vi "CRYGet Time Curve array.vi"(4 "Scaling":u16=1, 6 "Unit Info In":T5={"Y unit In"="dB", "dB ref In"=1.0, "Y unit Out"="dB", "dB ref Out"=1.0, "Y unit Curve"="dB", "dB ref Curve"=1.0, "Y data  Curve"=0, "Y data Time"=0}, 7 "Additive Info":T2, 8 "Harmonics array":dbl[](array[numeric]), 9 "Option Array In":bool[](array[boolean]), 10 "Averaging":u16, 11 "Algorithm":u16) -> (0 "Display Array":T3(array[cluster]), 1 "Unit Info Out":T4[](array[typedef]), 2 "Curve Info Array Out":T1)   [LabVIEW 2013]
uses:
  Typedef Control/CRYUnit Info Cluster.ctl
  Typedef Control/CRYUnit Info Out Cluster.ctl
  Typedef Control/CRYAnalysis CurveName Cluster.ctl
panel:
  in  "Is Impedance?":bool
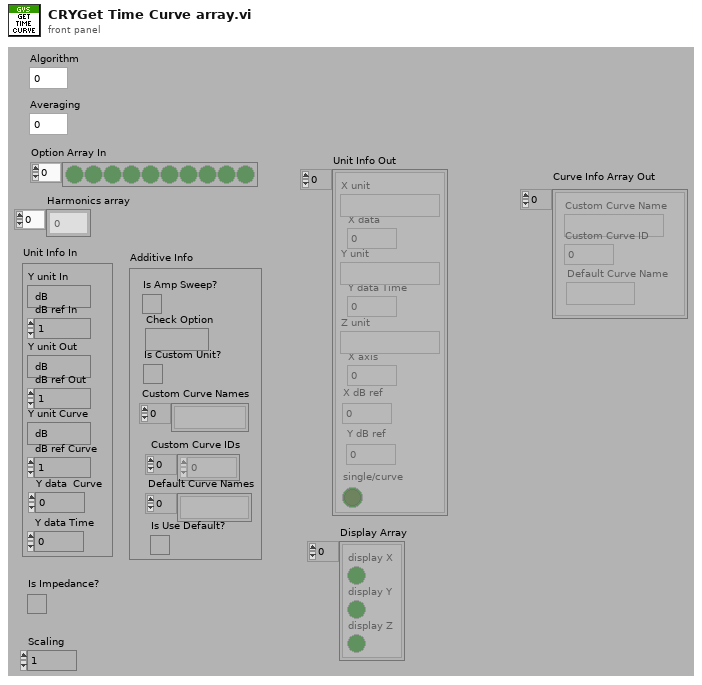
[diagram p1: front panel]
types:
  T1 = typedef "CRYAnalysis CurveName Cluster.ctl" = cluster{"Custom Curve Name":string, "Custom Curve ID":i32, "Default Curve Name":string}[]
  T2 = cluster{"Is Amp Sweep?":bool, "Check Option":string, "Is Custom Unit?":bool, "Custom Curve Names":string[], "Custom Curve IDs":i32[], "Default Curve Names":string[], "Is Use Default?":bool}
  T3 = cluster{"display X":bool, "display Y":bool, "display Z":bool}[]
  T4 = typedef "CRYUnit Info Out Cluster.ctl" = cluster{"X unit":string, "X data":u16, "Y unit":string, "Y data Time":u16, "Z unit":string, "X axis":u16, "X dB ref":dbl, "Y dB ref":dbl, "single/curve":bool}
  T5 = typedef "CRYUnit Info Cluster.ctl" = cluster{"Y unit In":string, "dB ref In":dbl, "Y unit Out":string, "dB ref Out":dbl, "Y unit Curve":string, "dB ref Curve":dbl, "Y data  Curve":u16, "Y data Time":u16}
  T6 = cluster{"display X":bool, "display Y":bool, "display Z":bool}
  T7 = enum32{"English", "Chinese", "Korean", "Japanese", "Russian", "Chinese traditional"}
  T8 = cluster{"X unit":string, "X data":u16, "Y unit In":string, "Scaling":u16, "Z unit":string, "X data":u16, "dB ref In":dbl, "dB ref In":dbl, "display X":bool}
  T9 = cluster{"X unit":string, "X data":u16, string, "Scaling":u16, "Z unit":string, "X data":u16, "dB ref In":dbl, "dB ref In":dbl, "display X":bool}
  T10 = cluster{"X unit":string, "X data":u16, string, "Scaling":u16, "Z unit":string, "X data":u16, "dB ref In":dbl, "dB ref In":dbl, "display X":bool}[]
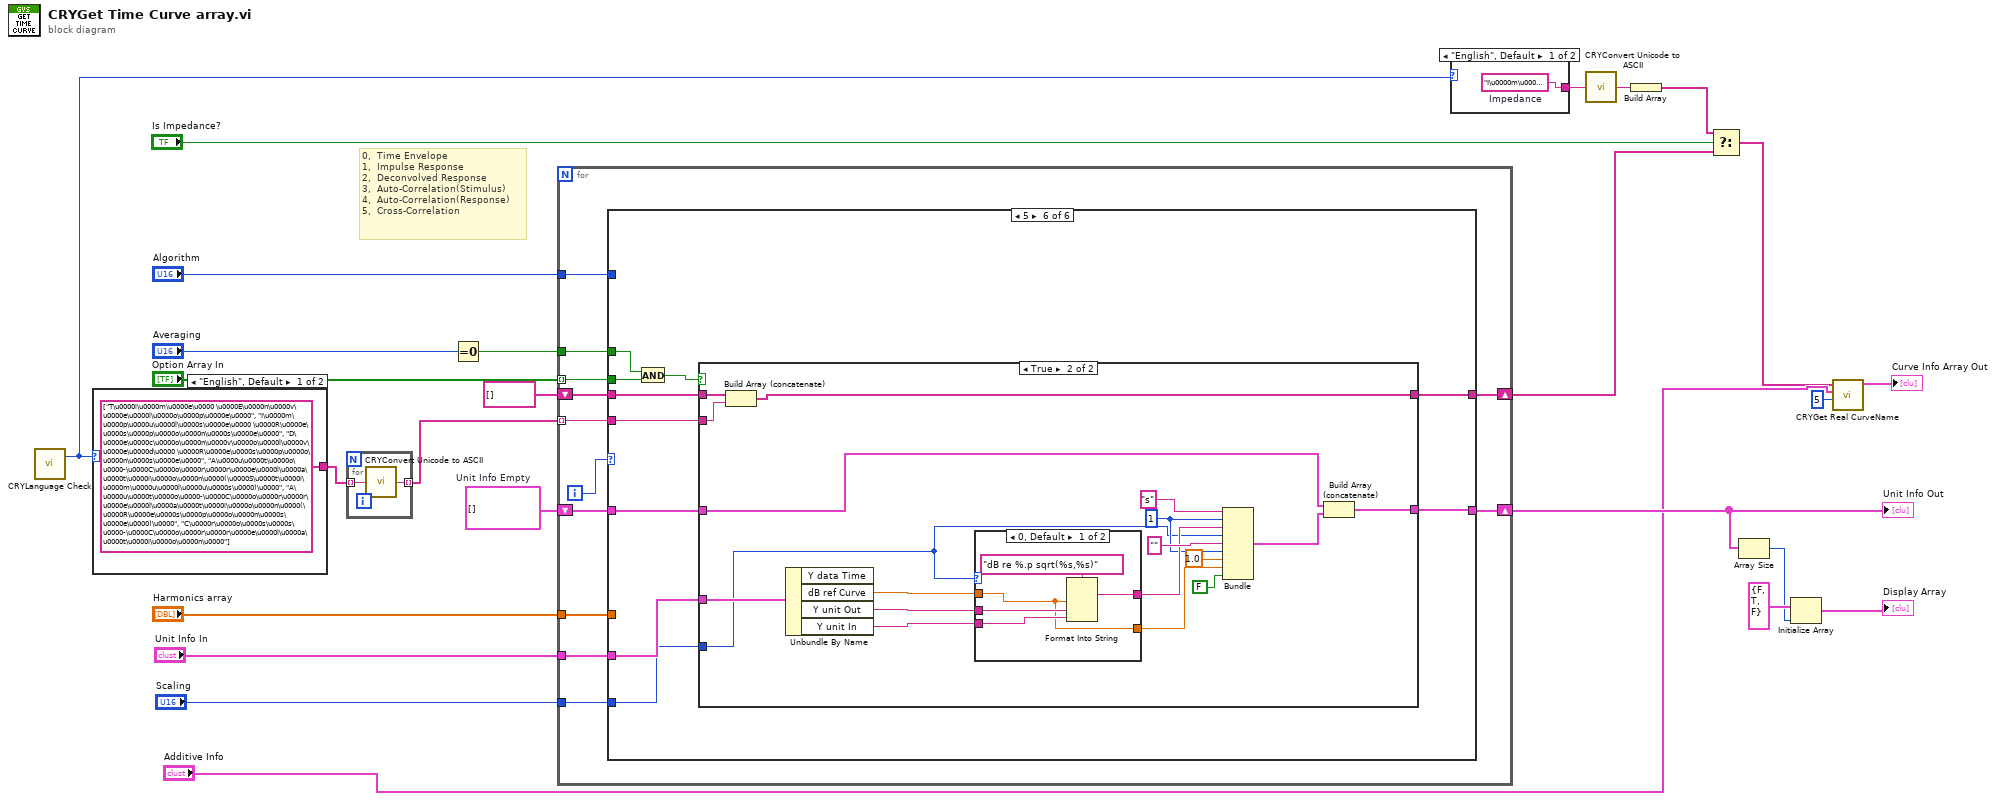
[diagram p0: block diagram]
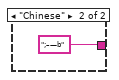
[diagram p2: hidden frame]
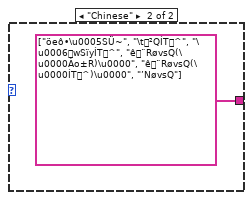
[diagram p3: hidden frame]
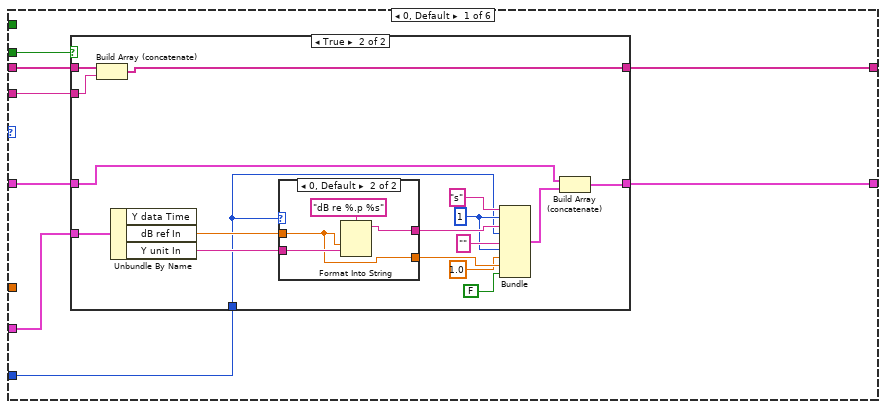
[diagram p4: hidden frame]
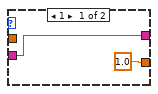
[diagram p6: hidden frame]
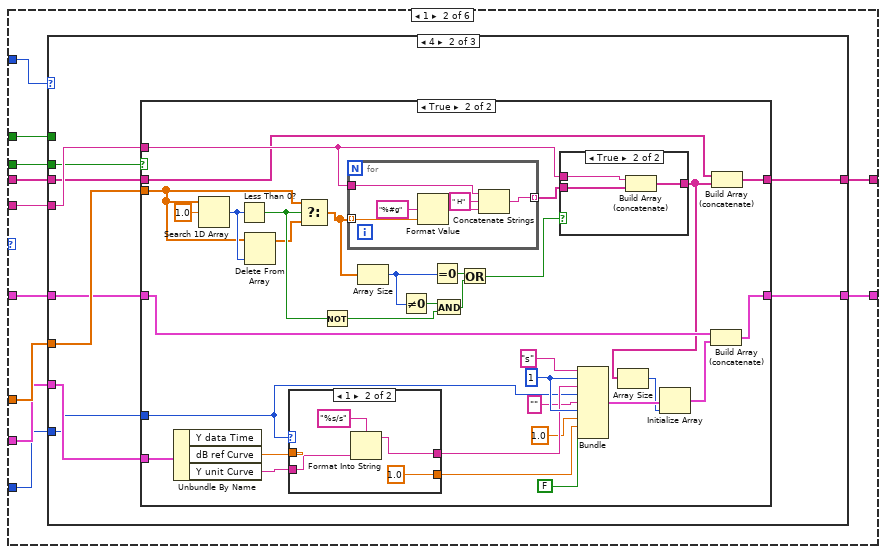
[diagram p7: hidden frame]
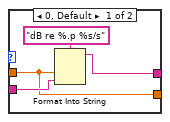
[diagram p10: hidden frame]
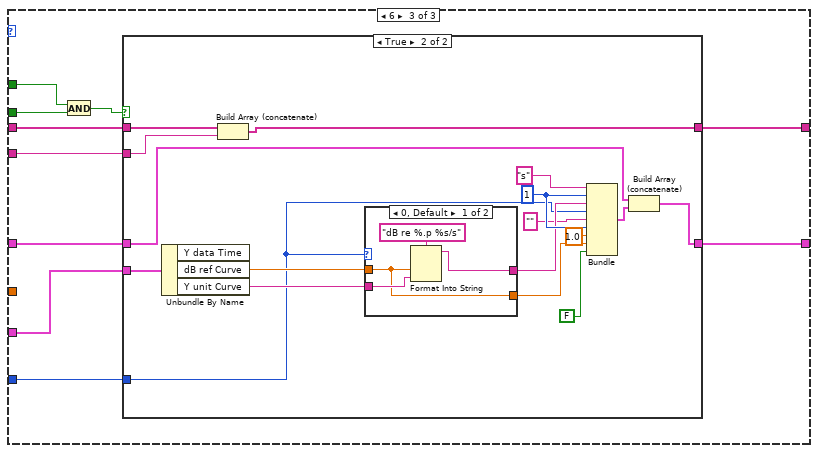
[diagram p12: hidden frame]
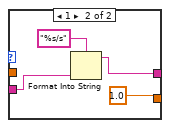
[diagram p14: hidden frame]
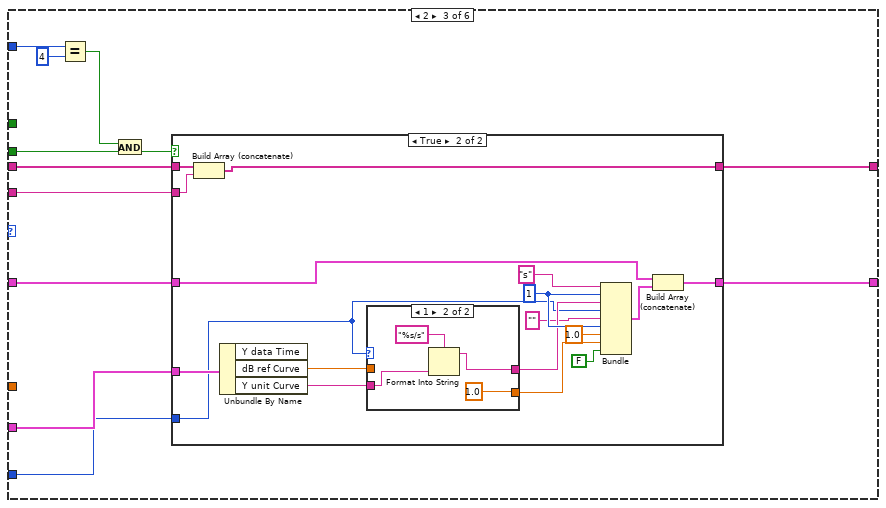
[diagram p15: hidden frame]
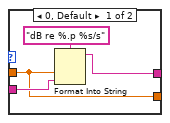
[diagram p17: hidden frame]
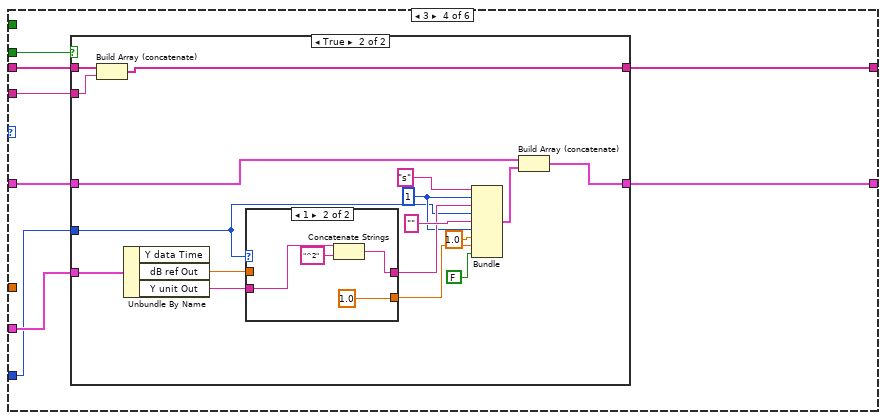
[diagram p18: hidden frame]
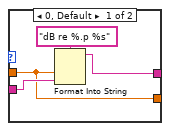
[diagram p20: hidden frame]
diagram:
  w15 = T4[] []  # Unit Info Empty
  # "0,  Time Envelope\n1,  Impulse Response\n2,  Deconvolved Response\n3,  Auto-Correlation(Stimulus)\n4,  Auto-Correlation(Response)\n5,  Cross-Correlation"
  n1 = call "CRYLanguage Check.vi"() -> ("Language"=w1:T7)  [unwired: 10 in, 1 out]
  n2 = case shown="\"English\", Default" w1 {
    tunnel: [string[] ["T\u0000i\u0000m\u0000e\u0000 \u0000E\u0000n\u0000v\u0000e\u0000l\u0000o\u0000p\u0000e\u0000", "I\u0000m\u0000p\u0000u\u0000l\u0000s\u0000e\u0000 \u0000R\u0000e\u0000s\u0000p\u0000o\u0000n\u0000s\u0000e\u0000", "D\u0000e\u0000c\u0000o\u0000n\u0000v\u0000o\u0000l\u0000v\u0000e\u0000d\u0000 \u0000R\u0000e\u0000s\u0000p\u0000o\u0000n\u0000s\u0000e\u0000", "A\u0000u\u0000t\u0000o\u0000-\u0000C\u0000o\u0000r\u0000r\u0000e\u0000l\u0000a\u0000t\u0000i\u0000o\u0000n\u0000(\u0000S\u0000t\u0000i\u0000m\u0000u\u0000l\u0000u\u0000s\u0000)\u0000", "A\u0000u\u0000t\u0000o\u0000-\u0000C\u0000o\u0000r\u0000r\u0000e\u0000l\u0000a\u0000t\u0000i\u0000o\u0000n\u0000(\u0000R\u0000e\u0000s\u0000p\u0000o\u0000n\u0000s\u0000e\u0000)\u0000", "C\u0000r\u0000o\u0000s\u0000s\u0000-\u0000C\u0000o\u0000r\u0000r\u0000e\u0000l\u0000a\u0000t\u0000i\u0000o\u0000n\u0000"] ("Array") string[] ["öeô•\u0005SÜ~", "\t²QÍT^", "\u0006wSïyÍT^", "ê¨RøvsQ(\u0000Ào±R)\u0000", "ê¨RøvsQ(\u0000ÍT^)\u0000", "’NøvsQ"] ("Array")] -> w5
    frame "English", Default {
    }
    frame "Chinese" {
    }
  }
  n3 = for {
    tunnel: w5 -> [w29] mode=indexing
    tunnel: [w28] -> w6 mode=indexing
    n4 = call "CRYConvert Unicode to ASCII.vi"("Unicode"=w29) -> ("ASCII"=w28:string)  [unwired: 4 in]
  }
  n5 = Equal To 0?(x="Averaging") -> (x = 0?=w23:bool)
  n6 = for {
    tunnel: w6 -> [w39] mode=indexing
    tunnel: "Option Array In" -> [w41] mode=indexing
    shift-right: [w38] -> w10
    shift-left: string[] [] ("Array") -> [w40]
    tunnel: w23 -> [w36]
    tunnel: "Algorithm" -> [w35]
    tunnel: "Harmonics array" -> [w34]
    tunnel: "Unit Info In" -> [w33]
    shift-right: [w32] -> w14
    shift-left: w15 -> [w31]
    tunnel: "Scaling" -> [w30]
    i -> [w37]
    n7 = case shown="5" w37 {
      tunnel: w41 -> [w49 w82 w195 w233 w268 w302]
      tunnel: w40 -> [w48 w85 w198 w232 w267 w305]
      tunnel: w39 -> [w47 w84 w197 w231 w266 w304]
      tunnel: [w46 w83 w196 w230 w265 w303] -> w38
      tunnel: w36 -> [_ w81 _ _ _ w301]
      tunnel: w35 -> [_ w80 w194 _ _ _]
      tunnel: w34 -> [_ w79 _ _ _ _]
      tunnel: w33 -> [w44 w76 w190 w228 w263 w297]
      tunnel: [w43 w78 w189 w227 w262 w298] -> w32
      tunnel: w31 -> [w45 w77 w188 w229 w264 w299]
      tunnel: w30 -> [w42 w75 w187 w226 w261 w296]
      frame 0, Default {
        n8 = case shown="True" w49 {
          tunnel: w48 -> [w51 w68]
          tunnel: w47 -> [_ w67]
          tunnel: [w51 w66] -> w46
          tunnel: w45 -> [w50 w57]
          tunnel: w44 -> [_ w58]
          tunnel: [w50 w56] -> w43
          tunnel: w42 -> [_ w53]
          frame False {
          }
          frame True {
            w62 = u16 1 ("X data")
            n9 = Build Array (concatenate)(w68, w67) -> (w66:string[])
            n10 = Unbundle By Name(w58) -> ("dB ref In"=w61:dbl, "Y unit In"=w60:string)  [unwired: 1 out]
            n11 = case shown="0, Default" w53 {
              tunnel: [w70 w72] -> w63
              tunnel: w61 -> [_ w71]
              tunnel: w60 -> [w70 w73]
              tunnel: [1.0 ("dB ref In") w71] -> w55
              frame 1 {
              }
              frame 0, Default {
                n12 = Format Into String(format string="dB re %.p %s", w71, w73) -> (resulting string=w72:string)  [unwired: 2 in, 1 out]
              }
            }
            n13 = Bundle("X unit"="s", "X data"=w62, "Y unit In"=w63, "Scaling"=w53, "Z unit"="", "X data"=w62, "dB ref In"=1.0, "dB ref In"=w55, "display X"=FALSE) -> (w59:T8)  [unwired: 1 in]
            n14 = Build Array (concatenate)(w57, w59) -> (w56:T4[])
          }
        }
      }
      frame 1 {
        n15 = case shown="4" w80 {
          tunnel: w85 -> [w87 w94 w159]
          tunnel: w84 -> [_ w95 w158]
          tunnel: [w87 w93 w157] -> w83
          tunnel: w82 -> [_ w92 w156]
          tunnel: w81 -> [_ _ w155]
          tunnel: w79 -> [_ w96 _]
          tunnel: [w86 w91 w153] -> w78
          tunnel: w77 -> [w86 w90 w152]
          tunnel: w76 -> [_ w89 w151]
          tunnel: w75 -> [_ w88 w150]
          frame Default {
          }
          frame 4 {
            n16 = case shown="True" w92 {
              tunnel: w96 -> [_ w119]
              tunnel: w95 -> [_ w118]
              tunnel: w94 -> [w98 w117]
              tunnel: [w98 w116] -> w93
              tunnel: [w97 w115] -> w91
              tunnel: w90 -> [w97 w114]
              tunnel: w89 -> [_ w107]
              tunnel: w88 -> [_ w100]
              frame False {
              }
              frame True {
                w111 = u16 1 ("X data")
                n17 = Unbundle By Name(w107) -> ("dB ref Curve"=w112:dbl, "Y unit Curve"=w113:string)  [unwired: 1 out]
                n18 = Search 1D Array(1D array=w119, element=1.0) -> (index of element=w121:i32)  [unwired: 1 out]
                n19 = Less Than 0?(x=w121) -> (x < 0?=w128:bool)
                n20 = Delete From Array(array=w119, index=w121) -> (array with subset deleted=w122:dbl[])  [unwired: 1 in, 1 out]
                n21 = case shown="1" w100 {
                  tunnel: [w133 w137] -> w110
                  tunnel: w112 -> [w132 _]
                  tunnel: w113 -> [w134 w139]
                  tunnel: [w132 1.0 ("dB ref In")] -> w101
                  frame 0, Default {
                    n22 = Format Into String(format string="dB re %.p %s/s", w132, w134) -> (resulting string=w133:string)  [unwired: 2 in, 1 out]
                  }
                  frame 1 {
                    n23 = Format Into String(format string="%s/s", w139) -> (resulting string=w137:string)  [unwired: 2 in, 1 out]
                  }
                }
                n24 = Select(t=w119, s=w128, f=w122) -> (s? t:f=w124:dbl[])
                n25 = Not(x=w128) -> (.not. x?=w129:bool)
                n26 = for {
                  tunnel: w124 -> [w148] mode=indexing
                  tunnel: [w146] -> w123 mode=indexing
                  tunnel: w118 -> [w145]
                  n27 = Format Value(format string="%#g", value (0)=w148) -> (output string=w147:string)  [unwired: 1 out]
                  n28 = Concatenate Strings(w145, " H" ("string"), w147) -> (w146:string)
                }
                n29 = Array Size(array=w124) -> (size(s)=w126:i32)
                n30 = Not Equal To 0?(x=w126) -> (x != 0?=w127:bool)
                n31 = Equal To 0?(x=w126) -> (x = 0?=w125:bool)
                n32 = And(x=w127, y=w129) -> (x .and. y?=w130:bool)
                n33 = Or(x=w125, y=w130) -> (x .or. y?=w131:bool)
                n34 = case shown="True" w131 {
                  tunnel: w123 -> [w140 w142]
                  tunnel: [w140 w141] -> w104
                  tunnel: w118 -> [_ w143]
                  frame False {
                  }
                  frame True {
                    n35 = Build Array (concatenate)(w143, w142) -> (w141:string[])
                  }
                }
                n36 = Bundle("X unit"="s", "X data"=w111, w110, "Scaling"=w100, "Z unit"="", "X data"=w111, "dB ref In"=1.0, "dB ref In"=w101, "display X"=FALSE) -> (w106:T9)  [unwired: 1 in]
                n37 = Array Size(array=w104) -> (size(s)=w105:i32)
                n38 = Initialize Array(w106, w105) -> (w103:T10)
                n39 = Build Array (concatenate)(w114, w103) -> (w115:T4[])
                n40 = Build Array (concatenate)(w117, w104) -> (w116:string[])
              }
            }
          }
          frame 6 {
            n41 = And(x=w155, y=w156) -> (x .and. y?=w154:bool)
            n42 = case shown="True" w154 {
              tunnel: w159 -> [w161 w178]
              tunnel: w158 -> [_ w176]
              tunnel: [w161 w177] -> w157
              tunnel: [w160 w174] -> w153
              tunnel: w152 -> [w160 w175]
              tunnel: w151 -> [_ w167]
              tunnel: w150 -> [_ w163]
              frame False {
              }
              frame True {
                w171 = u16 1 ("X data")
                n43 = Unbundle By Name(w167) -> ("dB ref Curve"=w172:dbl, "Y unit Curve"=w173:string)  [unwired: 1 out]
                n44 = Build Array (concatenate)(w178, w176) -> (w177:string[])
                n45 = case shown="0, Default" w163 {
                  tunnel: [w180 w184] -> w170
                  tunnel: w172 -> [w179 _]
                  tunnel: w173 -> [w181 w186]
                  tunnel: [w179 1.0 ("dB ref In")] -> w165
                  frame 0, Default {
                    n46 = Format Into String(format string="dB re %.p %s/s", w179, w181) -> (resulting string=w180:string)  [unwired: 2 in, 1 out]
                  }
                  frame 1 {
                    n47 = Format Into String(format string="%s/s", w186) -> (resulting string=w184:string)  [unwired: 2 in, 1 out]
                  }
                }
                n48 = Bundle("X unit"="s", "X data"=w171, w170, "Scaling"=w163, "Z unit"="", "X data"=w171, "dB ref In"=1.0, "dB ref In"=w165, "display X"=FALSE) -> (w166:T9)  [unwired: 1 in]
                n49 = Build Array (concatenate)(w175, w166) -> (w174:T4[])
              }
            }
          }
        }
      }
      frame 2 {
        n50 = Equal?(x=w194, y=u16 4) -> (x = y?=w191:bool)
        n51 = And(x=w191, y=w195) -> (x .and. y?=w192:bool)
        n52 = case shown="True" w192 {
          tunnel: w198 -> [w200 w217]
          tunnel: w197 -> [_ w215]
          tunnel: [w200 w216] -> w196
          tunnel: w190 -> [_ w208]
          tunnel: [w199 w207] -> w189
          tunnel: w188 -> [w199 w206]
          tunnel: w187 -> [_ w202]
          frame False {
          }
          frame True {
            w212 = u16 1 ("X data")
            n53 = Build Array (concatenate)(w217, w215) -> (w216:string[])
            n54 = Unbundle By Name(w208) -> ("dB ref Curve"=w213:dbl, "Y unit Curve"=w214:string)  [unwired: 1 out]
            n55 = case shown="1" w202 {
              tunnel: [w219 w223] -> w211
              tunnel: w213 -> [w218 _]
              tunnel: w214 -> [w220 w225]
              tunnel: [w218 1.0 ("dB ref In")] -> w204
              frame 0, Default {
                n56 = Format Into String(format string="dB re %.p %s/s", w218, w220) -> (resulting string=w219:string)  [unwired: 2 in, 1 out]
              }
              frame 1 {
                n57 = Format Into String(format string="%s/s", w225) -> (resulting string=w223:string)  [unwired: 2 in, 1 out]
              }
            }
            n58 = Bundle("X unit"="s", "X data"=w212, w211, "Scaling"=w202, "Z unit"="", "X data"=w212, "dB ref In"=1.0, "dB ref In"=w204, "display X"=FALSE) -> (w205:T9)  [unwired: 1 in]
            n59 = Build Array (concatenate)(w206, w205) -> (w207:T4[])
          }
        }
      }
      frame 3 {
        n60 = case shown="True" w233 {
          tunnel: w232 -> [w235 w252]
          tunnel: w231 -> [_ w251]
          tunnel: [w235 w250] -> w230
          tunnel: w229 -> [w234 w240]
          tunnel: w228 -> [_ w243]
          tunnel: [w234 w241] -> w227
          tunnel: w226 -> [_ w237]
          frame False {
          }
          frame True {
            w246 = u16 1 ("X data")
            n61 = Build Array (concatenate)(w252, w251) -> (w250:string[])
            n62 = Unbundle By Name(w243) -> ("dB ref Out"=w245:dbl, "Y unit Out"=w244:string)  [unwired: 1 out]
            n63 = case shown="1" w237 {
              tunnel: [w254 w257] -> w247
              tunnel: w245 -> [w253 _]
              tunnel: w244 -> [w255 w259]
              tunnel: [w253 1.0 ("dB ref In")] -> w239
              frame 0, Default {
                n64 = Format Into String(format string="dB re %.p %s", w253, w255) -> (resulting string=w254:string)  [unwired: 2 in, 1 out]
              }
              frame 1 {
                n65 = Concatenate Strings(w259, "^2" ("string")) -> (w257:string)
              }
            }
            n66 = Bundle("X unit"="s", "X data"=w246, w247, "Scaling"=w237, "Z unit"="", "X data"=w246, "dB ref In"=1.0, "dB ref In"=w239, "display X"=FALSE) -> (w242:T9)  [unwired: 1 in]
            n67 = Build Array (concatenate)(w240, w242) -> (w241:T4[])
          }
        }
      }
      frame 4 {
        n68 = case shown="True" w268 {
          tunnel: w267 -> [w270 w287]
          tunnel: w266 -> [_ w286]
          tunnel: [w270 w285] -> w265
          tunnel: w264 -> [w269 w275]
          tunnel: w263 -> [_ w276]
          tunnel: [w269 w277] -> w262
          tunnel: w261 -> [_ w272]
          frame False {
          }
          frame True {
            w281 = u16 1 ("X data")
            n69 = Build Array (concatenate)(w287, w286) -> (w285:string[])
            n70 = Unbundle By Name(w276) -> ("dB ref In"=w280:dbl, "Y unit In"=w279:string)  [unwired: 1 out]
            n71 = case shown="1" w272 {
              tunnel: [w289 w292] -> w282
              tunnel: w280 -> [w288 _]
              tunnel: w279 -> [w290 w293]
              tunnel: [w288 1.0 ("dB ref In")] -> w274
              frame 0, Default {
                n72 = Format Into String(format string="dB re %.p %s", w288, w290) -> (resulting string=w289:string)  [unwired: 2 in, 1 out]
              }
              frame 1 {
                n73 = Concatenate Strings(w293, "^2" ("string")) -> (w292:string)
              }
            }
            n74 = Bundle("X unit"="s", "X data"=w281, w282, "Scaling"=w272, "Z unit"="", "X data"=w281, "dB ref In"=1.0, "dB ref In"=w274, "display X"=FALSE) -> (w278:T9)  [unwired: 1 in]
            n75 = Build Array (concatenate)(w275, w278) -> (w277:T4[])
          }
        }
      }
      frame 5 {
        n76 = And(x=w301, y=w302) -> (x .and. y?=w300:bool)
        n77 = case shown="True" w300 {
          tunnel: w305 -> [w307 w325]
          tunnel: w304 -> [_ w323]
          tunnel: [w307 w324] -> w303
          tunnel: w299 -> [w306 w322]
          tunnel: [w306 w321] -> w298
          tunnel: w297 -> [_ w313]
          tunnel: w296 -> [_ w309]
          frame False {
          }
          frame True {
            w316 = u16 1 ("X data")
            n78 = Build Array (concatenate)(w325, w323) -> (w324:string[])
            n79 = Unbundle By Name(w313) -> ("dB ref Curve"=w315:dbl, "Y unit Out"=w314:string, "Y unit In"=w320:string)  [unwired: 1 out]
            n80 = case shown="0, Default" w309 {
              tunnel: [w329 w332] -> w317
              tunnel: w315 -> [w326 _]
              tunnel: w314 -> [w328 w334]
              tunnel: w320 -> [w327 w333]
              tunnel: [w326 1.0 ("dB ref In")] -> w311
              frame 0, Default {
                n81 = Format Into String(format string="dB re %.p sqrt(%s,%s)", w326, w328, w327) -> (resulting string=w329:string)  [unwired: 2 in, 1 out]
              }
              frame 1 {
                n82 = Format Into String(format string="%s,%s", w334, w333) -> (resulting string=w332:string)  [unwired: 2 in, 1 out]
              }
            }
            n83 = Bundle("X unit"="s", "X data"=w316, w317, "Scaling"=w309, "Z unit"="", "X data"=w316, "dB ref In"=1.0, "dB ref In"=w311, "display X"=FALSE) -> (w312:T9)  [unwired: 1 in]
            n84 = Build Array (concatenate)(w322, w312) -> (w321:T4[])
          }
        }
      }
    }
  }
  "Unit Info Out" <- w14
  n85 = case shown="\"English\", Default" w1 {
    tunnel: [w336 ";–—b" ("Unicode")] -> w3
    frame "English", Default {
      w336 = "I\u0000m\u0000p\u0000e\u0000d\u0000an\u0000c\u0000e\u0000"  # Impedance
    }
    frame "Chinese" {
    }
  }
  n86 = call "CRYConvert Unicode to ASCII.vi"("Unicode"=w3) -> ("ASCII"=w2:string)  [unwired: 4 in]
  n87 = Build Array(w2) -> (w4:string[])
  n88 = Select(t=w4, s="Is Impedance?", f=w10) -> (s? t:f=w9:string[])
  n89 = Array Size(array=w14) -> (size(s)=w16:i32)
  n90 = Initialize Array(T6 {"display X"=FALSE, "display Y"=TRUE, "display Z"=FALSE}, w16) -> (→"Display Array":T3)
  n91 = call "CRYGet Real CurveName.vi"("Key No"=5, "Additive Info"="Additive Info", "CurveArrayByType"=w9) -> ("Curve Info Array Out"=→"Curve Info Array Out":T1)  [unwired: 8 in]
